vi "Add Item.vi"(8 "error in (no error)":errorcluster, 10 "ItemInfo":T1={"Parent Tag (\"\")"="", "Child Position (-1=End)"=-1, "Left Cell String (\"\" = Same as Child Tag)"="", "Child Text[]"=[], "Child Tag"="", "Child Only? (F)"=FALSE}, 11 "Tree in":refnum<class "TreeControl.lvclass">) -> (0 "error out":errorcluster, 2 "Add Item Tag":string, 3 "Tree (dup)":refnum<class "TreeControl.lvclass">)   [LabVIEW 2015, in "TreeControl.lvclass"]
doc: "<b> </b> <b> </b>\n©2016 Q Software Innovations, LLC (QSI)\nwritten by Quentin Alldredge\nproduced in LabVIEW 2015\n\nsupport@qsoftwareinnovations.com\nwww.qsoftwareinnovations.com\n\nAll rights reserved.\n\nRedistribution and use in source and binary forms, with or without modification, are permitted provided that the following conditions are met:\n\n * Redistributions of source code must retain the above copyright notice, this list of conditions and the following disclaimer.\n * Redistributions in binary form must reproduce the above copyright notice, this list of conditions and the following disclaimer in the documentation and/or other materials provided with the distribution.\n * Neither the name of Q Software Innovations, LLC. nor the names of its contributors may be used to endorse or promote products derived from this software without specific prior written permission.\n\nTHIS SOFTWARE IS PROVIDED BY THE COPYRIGHT HOLDERS AND CONTRIBUTORS \"AS IS\" AND ANY EXPRESS OR IMPLIED WARRANTIES, INCLUDING, BUT NOT LIMITED TO, THE IMPLIED WARRANTIES OF MERCHANTABILITY AND FITNESS FOR A PARTICULAR PURPOSE ARE DISCLAIMED. IN NO EVENT SHALL THE COPYRIGHT OWNER OR CONTRIBUTORS BE LIABLE FOR ANY DIRECT, INDIRECT, INCIDENTAL, SPECIAL, EXEMPLARY, OR CONSEQUENTIAL DAMAGES (INCLUDING, BUT NOT LIMITED TO, PROCUREMENT OF SUBSTITUTE GOODS OR SERVICES; LOSS OF USE, DATA, OR PROFITS; OR BUSINESS INTERRUPTION) HOWEVER CAUSED AND ON ANY THEORY OF LIABILITY, WHETHER IN CONTRACT, STRICT LIABILITY, OR TORT (INCLUDING NEGLIGENCE OR OTHERWISE) ARISING IN ANY WAY OUT OF THE USE OF THIS SOFTWARE, EVEN IF ADVISED OF THE POSSIBILITY OF SUCH DAMAGE."
uses:
  TreeControl.lvclass
  Add Item Info Cluster.ctl
  TreeControl.lvclass/TreeControl.ctl
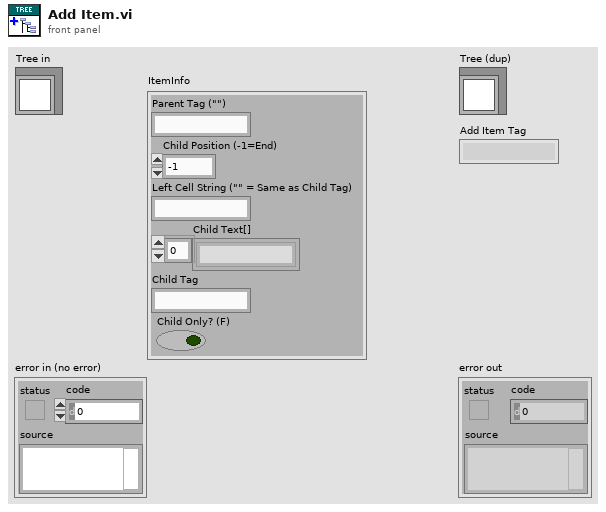
[diagram p1: front panel]
types:
  T1 = typedef "TreeControl.lvclass/Add Item Info Cluster.ctl" = cluster{"Parent Tag (\"\")":string, "Child Position (-1=End)":i32, "Left Cell String (\"\" = Same as Child Tag)":string, "Child Text[]":string[], "Child Tag":string, "Child Only? (F)":bool}
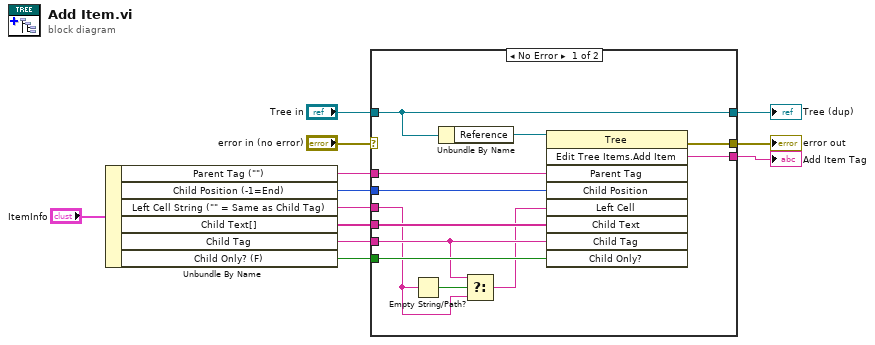
[diagram p0: block diagram]
diagram:
  n1 = Unbundle By Name("ItemInfo") -> ("Parent Tag (\"\")"=w6:string, "Child Position (-1=End)"=w5:i32, "Left Cell String (\"\" = Same as Child Tag)"=w4:string, "Child Text[]"=w3:string[], "Child Tag"=w2:string, "Child Only? (F)"=w1:bool)
  n2 = case shown="No Error" "error in (no error)" {
    selector: "error in (no error)" -> [_ w26]
    tunnel: [w24 w26] -> w11
    tunnel: [w14 w25] -> w9
    tunnel: "Tree in" -> [w14 w25]
    tunnel: [w23 _] -> w8
    tunnel: w6 -> [w22 _]
    tunnel: w5 -> [w21 _]
    tunnel: w4 -> [w16 _]
    tunnel: w3 -> [w20 _]
    tunnel: w2 -> [w17 _]
    tunnel: w1 -> [w19 _]
    frame No Error {
      n3 = Empty String/Path?(string/path=w16) -> (empty?=w18:bool)
      n4 = Unbundle By Name(w14) -> ("Reference"=w13:refnum<vi>)
      n5 = Select(t=w17, s=w18, f=w16) -> (s? t:f=w15:string)
      n6 = invoke on="Invoke Node" class="Tree" method="Edit Tree Items.Add Item"(reference=w13, "Parent Tag"=w22, "Child Position"=w21, "Left Cell"=w15, "Child Text"=w20, "Child Tag"=w17, "Child Only?"=w19) -> (error out=w24:errorcluster, "Edit Tree Items:Add Item"=w23:string)  [unwired: 2 in, 7 out]
    }
    frame Error {
    }
  }
  "error out" <- w11
  "Tree (dup)" <- w9
  "Add Item Tag" <- w8
